vi "S2DS_Change Data save info.vi"(2 "error in (no error)":errorcluster, 3 "Data saving info":T1={"File path"=path "", "Header"="", "File name"="", "False channel"=[], "Channel names"=[], "Buffer size"=0, "Format"="%.6f"}) -> (0 "error out":errorcluster, 1 "Data saving info 2":T1={"File path"=path "", "Header"="", "File name"="", "False channel"=[], "Channel names"=[], "Buffer size"=0, "Format"="%.6f"})   [LabVIEW 2025]
uses:
  TYPE DEFS/S2DS_Data saving info.ctl
  <vilib>/Utility/config.llb/Read Key (U32).vi
  <vilib>/Utility/config.llb/Read Key (Path).vi
  <vilib>/Utility/config.llb/Write Key (Path).vi
  <vilib>/Utility/config.llb/Write Key (I32).vi
  <vilib>/Utility/config.llb/NI_LVConfig.lvlib
panel:
  in  "Logbook path":path
  in  "File tag":string
  in  "File No":i32
  in  "Header":string
  in  "Format":string(combo)="%.6f"
  in  "Buffer size":i32
  in  "EXIT":bool
  # "Edit data save info..."
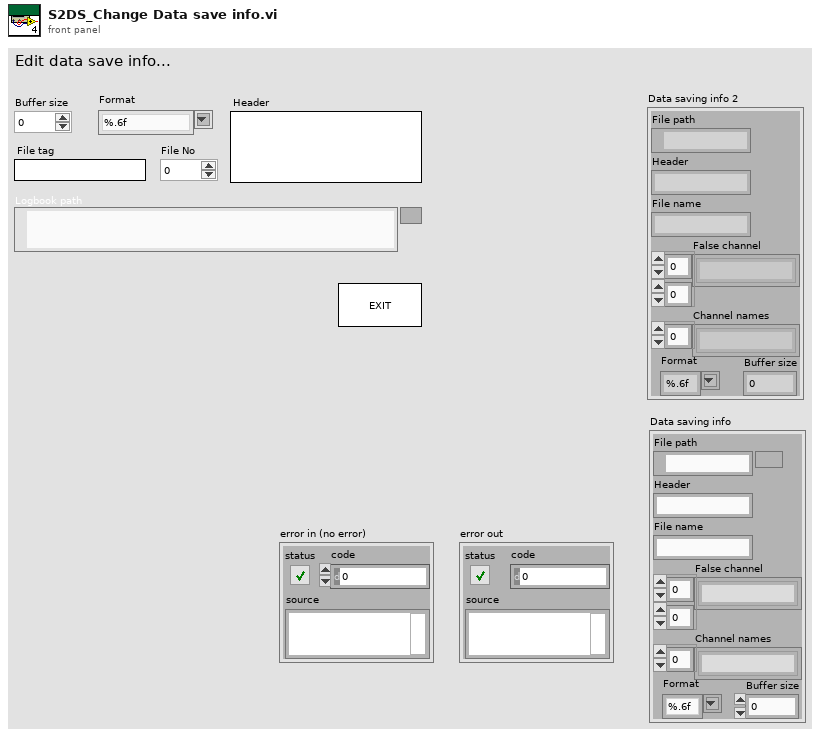
[diagram p1: front panel]
types:
  T1 = typedef "S2DS_Data saving info.ctl" = cluster{"File path":path, "Header":string, "File name":string, "False channel":string[][], "Channel names":string[], "Buffer size":i32, "Format":string}
  T2 = typedef "NI_LVConfig.lvlib/Config Data RefNum.ctl" = refnum<k1>
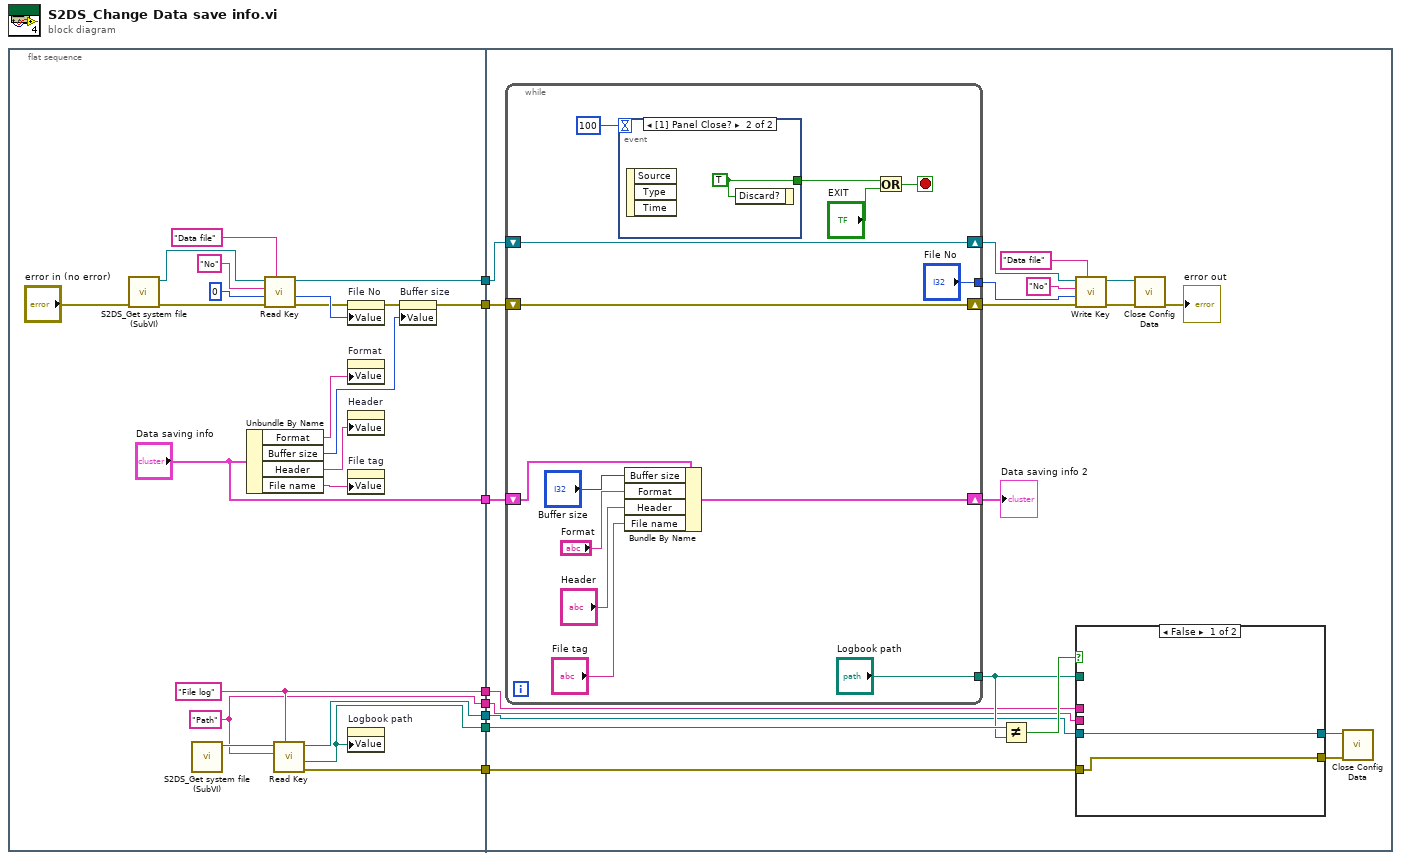
[diagram p0: block diagram]
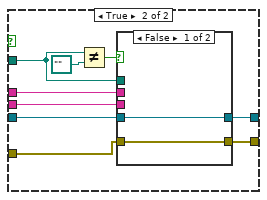
[diagram p2: hidden frame]
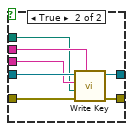
[diagram p3: hidden frame]
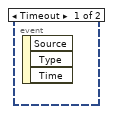
[diagram p4: hidden frame]
diagram:
  n1 = flat-sequence {
    tunnel: ["Data saving info"] -> w8
    tunnel: [w17] -> w7
    tunnel: [w16] -> w6
    tunnel: [w13] -> w5
    tunnel: [w12] -> w4
    tunnel: [w11] -> w3
    tunnel: [w10] -> w2
    tunnel: [w9] -> w1
    tunnel: w8 -> [w51]
    tunnel: w7 -> [w49]
    tunnel: w6 -> [w45]
    tunnel: w5 -> [w39]
    tunnel: w4 -> [w36]
    tunnel: w3 -> [w35]
    tunnel: w2 -> [w34]
    tunnel: w1 -> [w33]
    frame #0 {
      w9 = "Path" ("key")
      w10 = "File log" ("section")
      n2 = call "S2DS_Get system file (SubVI).vi"("error in (no error)"="error in (no error)") -> ("error out"=w20:errorcluster, "Refnum out"=w22:T2)  [unwired: 9 in]
      n3 = call "S2DS_Get system file (SubVI).vi"() -> ("Refnum out"=w14:T2)  [unwired: 10 in, 1 out]
      n4 = Unbundle By Name("Data saving info") -> ("Format"=w28:string, "Buffer size"=w29:i32, "Header"=w27:string, "File name"=w15:string)
      n5 = call-poly <vilib>:"Read Key.vi"("section"="Data file", "error in (no error)"=w20, "default value"=u32 0, "key"="No", "refnum"=w22) -> ("error out"=w19:errorcluster, "value"=w21:u32, "refnum out"=w17:T2)  [unwired: 3 in, 1 out]
      n6 = call-poly <vilib>:"Read Key.vi"("section"=w10, "key"=w9, "refnum"=w14) -> ("error out"=w11:errorcluster, "value"=w13:path, "refnum out"=w12:T2)  [unwired: 5 in, 1 out]
      n7 = property on="File No" class="DigNum (strict)"(error in=w19, "Value"=w21) -> (error out=w18:errorcluster)  [unwired: 1 in, 1 out]
      n8 = property on="Format" class="CmbBox"("Value"=w28) -> ()  [unwired: 2 in, 2 out]
      n9 = property on="Header" class="Str"("Value"=w27) -> ()  [unwired: 2 in, 2 out]
      n10 = property on="File tag" class="Str"("Value"=w15) -> ()  [unwired: 2 in, 2 out]
      n11 = property on="Logbook path" class="Path"("Value"=w13) -> ()  [unwired: 2 in, 2 out]
      n12 = property on="Buffer size" class="DigNum (strict)"(error in=w18, "Value"=w29) -> (error out=w16:errorcluster)  [unwired: 1 in, 1 out]
    }
    frame #1 {
      n13 = while {
        shift-right: [w80] -> w50
        shift-left: w51 -> [w81]
        shift-right: [w76] -> w46
        shift-left: w49 -> [w76]
        shift-right: [w75] -> w44
        shift-left: w45 -> [w75]
        tunnel: ["File No"] -> w40
        tunnel: ["Logbook path"] -> w37
        stop <- w82 stop-if-true
        n14 = event shown="[1] Panel Close?" {
          selector: _ -> [_ _]
          dyn-events: _ -> [_ _]
          timeout: 100 -> [_ _]
          tunnel: [_ w86] -> w83
          event Timeout {
            n15 = event-data() -> ()  [unwired: 1 in, 3 out]
          }
          event Panel Close? {
            w86 = TRUE ("Discard?")
            n16 = event-data() -> ()  [unwired: 1 in, 3 out]
            n17 = event-data("Discard?"=w86) -> ()  [unwired: 1 in, 1 out]
          }
        }
        n18 = Bundle By Name(cluster=w81, "Buffer size"="Buffer size", "Format"="Format", "Header"="Header", "File name"="File tag") -> (w80:T1)
        n19 = Or(x=w83, y="EXIT") -> (x .or. y?=w82:bool)
      }
      "Data saving info 2" <- w50
      n20 = Not Equal?(x=w39, y=w37) -> (x != y?=w38:bool)
      n21 = call-poly <vilib>:"Write Key.vi"("section"="Data file", "error in (no error)"=w44, "value"=w40, "key"="No", "refnum"=w46) -> ("error out"=w42:errorcluster, "refnum out"=w43:T2)  [unwired: 4 in, 1 out]
      n22 = case shown="False" w38 {
        tunnel: w37 -> [_ w56]
        tunnel: w36 -> [w52 w60]
        tunnel: w35 -> [w53 w59]
        tunnel: w34 -> [_ w58]
        tunnel: w33 -> [_ w57]
        tunnel: [w53 w55] -> w32
        tunnel: [w52 w54] -> w31
        frame False {
        }
        frame True {
          n23 = Not Equal?(x=w56, y=path "") -> (x != y?=w61:bool)
          n24 = case shown="False" w61 {
            tunnel: w60 -> [w63 w71]
            tunnel: w59 -> [w64 w70]
            tunnel: w58 -> [_ w69]
            tunnel: w57 -> [_ w68]
            tunnel: w56 -> [_ w67]
            tunnel: [w64 w66] -> w55
            tunnel: [w63 w65] -> w54
            frame False {
            }
            frame True {
              n25 = call-poly <vilib>:"Write Key.vi"("section"=w69, "error in (no error)"=w70, "value"=w67, "key"=w68, "refnum"=w71) -> ("error out"=w66:errorcluster, "refnum out"=w65:T2)  [unwired: 4 in, 1 out]
            }
          }
        }
      }
      n26 = call <vilib>:"Close Config Data.vi"("error in (no error)"=w42, "refnum"=w43) -> ("error out"=→"error out":errorcluster)  [unwired: 8 in, 1 out]
      n27 = call <vilib>:"Close Config Data.vi"("error in (no error)"=w32, "refnum"=w31) -> ()  [unwired: 8 in, 2 out]
    }
  }
